vi "IntermediateBotLogic.vi"(8 "error in (no error)":errorcluster, 10 "Current Player":T1, 11 "Gameboard":T2) -> (0 "error out":errorcluster, 3 "Selected Index":i8)   [LabVIEW 2020]
uses:
  controls/Gameboard Data.ctl
  controls/Player.ctl
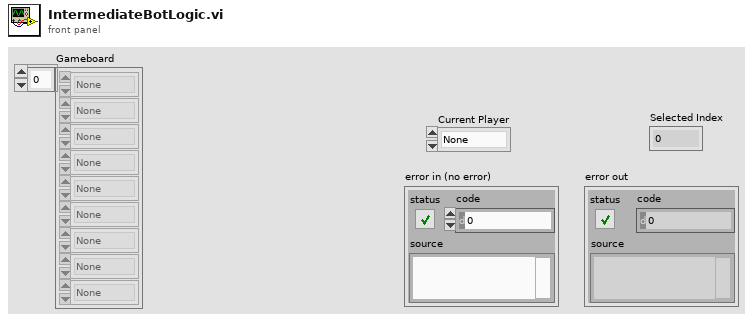
[diagram p1: front panel]
types:
  T1 = typedef "Player.ctl" = enum16{"None", "Player 1", "Player 2"}
  T2 = typedef "Gameboard Data.ctl" = enum16{"None", "Player 1", "Player 2"}[]
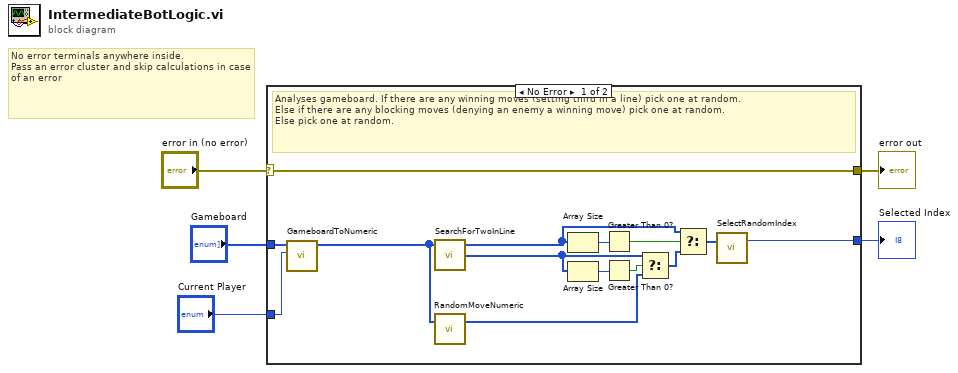
[diagram p0: block diagram]
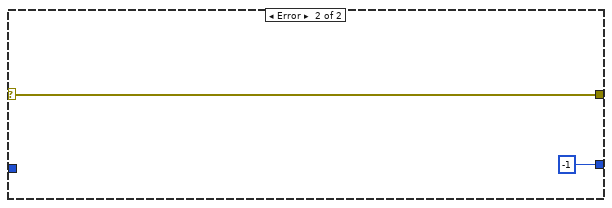
[diagram p2: hidden frame]
diagram:
  # "No error terminals anywhere inside.\nPass an error cluster and skip calculations in case of an error"
  n1 = case shown="No Error" "error in (no error)" {
    selector: "error in (no error)" -> [w13 w20]
    tunnel: "Gameboard" -> [w19 _]
    tunnel: "Current Player" -> [w18 _]
    tunnel: [w14 i8 -1 ("Selected Index")] -> w3
    tunnel: [w13 w20] -> w1
    frame No Error {
      # "Analyses gameboard. If there are any winning moves (setting third in a line) pick one at random. \nElse if there are any blocking moves (denying an enemy a winning move) pick one at random. \nElse pick one at random."
      n2 = call "GameboardToNumeric.vi"("CurrentPlayer"=w18, "Gameboard"=w19) -> ("NumericGameboard"=w15:i8[])  [unwired: 9 in]
      n3 = call "SearchForTwoInLine.vi"("NumericGameboard"=w15) -> ("Blocking Indices"=w8:i8[], "Wining Indices"=w10:i8[])  [unwired: 3 in]
      n4 = call "RandomMoveNumeric.vi"("NumericGameboard"=w15) -> ("Indices"=w7:i8[])  [unwired: 2 in]
      n5 = Array Size(array=w10) -> (size(s)=w17:i32)
      n6 = Array Size(array=w8) -> (size(s)=w16:i32)
      n7 = Greater Than 0?(x=w17) -> (x > 0?=w11:bool)
      n8 = Greater Than 0?(x=w16) -> (x > 0?=w9:bool)
      n9 = Select(t=w8, s=w9, f=w7) -> (s? t:f=w12:i8[])
      n10 = Select(t=w10, s=w11, f=w12) -> (s? t:f=w6:i8[])
      n11 = call "SelectRandomIndex.vi"("Indices"=w6) -> ("Selected Index"=w14:i8)  [unwired: 2 in]
    }
    frame Error {
    }
  }
  "Selected Index" <- w3
  "error out" <- w1
